vi "Blue Event Log Viewer Main.vi"() -> ()   [LabVIEW 2020, in "Blue Event Log Viewer.lvlib"]
uses:
  Blue Event Log Viewer.lvlib
  <userlib>/Blue Origin/Blue Event Log OpenSource/SubVIs/runlog logging levels.ctl
  <userlib>/Blue Origin/Blue Event Log OpenSource/SubVIs/runlog init options.ctl
  <userlib>/Blue Origin/Blue Event Log OpenSource/SubVIs/VisibleLogLevels.ctl
  <userlib>/Blue Origin/Blue Event Log OpenSource/Classes/RunLog/BlueEventLog.lvclass/BlueEventLog.ctl
  <userlib>/Blue Origin/Blue Event Log OpenSource/Classes/RunLog/Shutdown.vi
  <userlib>/Blue Origin/Blue Event Log OpenSource/SubVIs/Create WaitForFinish Notifier.vi
  <userlib>/Blue Origin/Blue Event Log OpenSource/SubVIs/WaitOn WaitForFinish Notifier.vi
  <userlib>/Blue Origin/Blue Event Log OpenSource/Classes/RunLog/Read Queue Validity.vi
  <vilib>/Utility/error.llb/Clear Errors.vi
  <userlib>/Blue Origin/Blue Event Log OpenSource/Classes/RunLog/New.vi
  <userlib>/Blue Origin/Blue Event Log OpenSource/Classes/RunLog/Stop Load Stream.vi
  <userlib>/Blue Origin/Blue Event Log OpenSource/Classes/RunLog/Clear.vi
  <vilib>/Utility/libraryn.llb/Check if File or Folder Exists.vi
  <vilib>/Utility/file.llb/Is Path and Not Empty.vi
  <vilib>/Utility/libraryn.llb/Librarian Path Location.vi
  <userlib>/_OpenG.lib/file/file.llb/File Exists__ogtk.vi
  <userlib>/_OpenG.lib/file/file.llb/File Exists - Scalar__ogtk.vi
  <userlib>/Blue Origin/Blue Event Log OpenSource/Classes/RunLog/Load log.vi
  <userlib>/Blue Origin/Blue Event Log OpenSource/Classes/RunLog/BlueEventLog.lvclass
  <userlib>/Blue Origin/Blue Event Log OpenSource/BlueEventLog_OpenSource.lvlib
panel:
  in  "Path":path
  in  "poll?":bool=TRUE caption="Poll?"
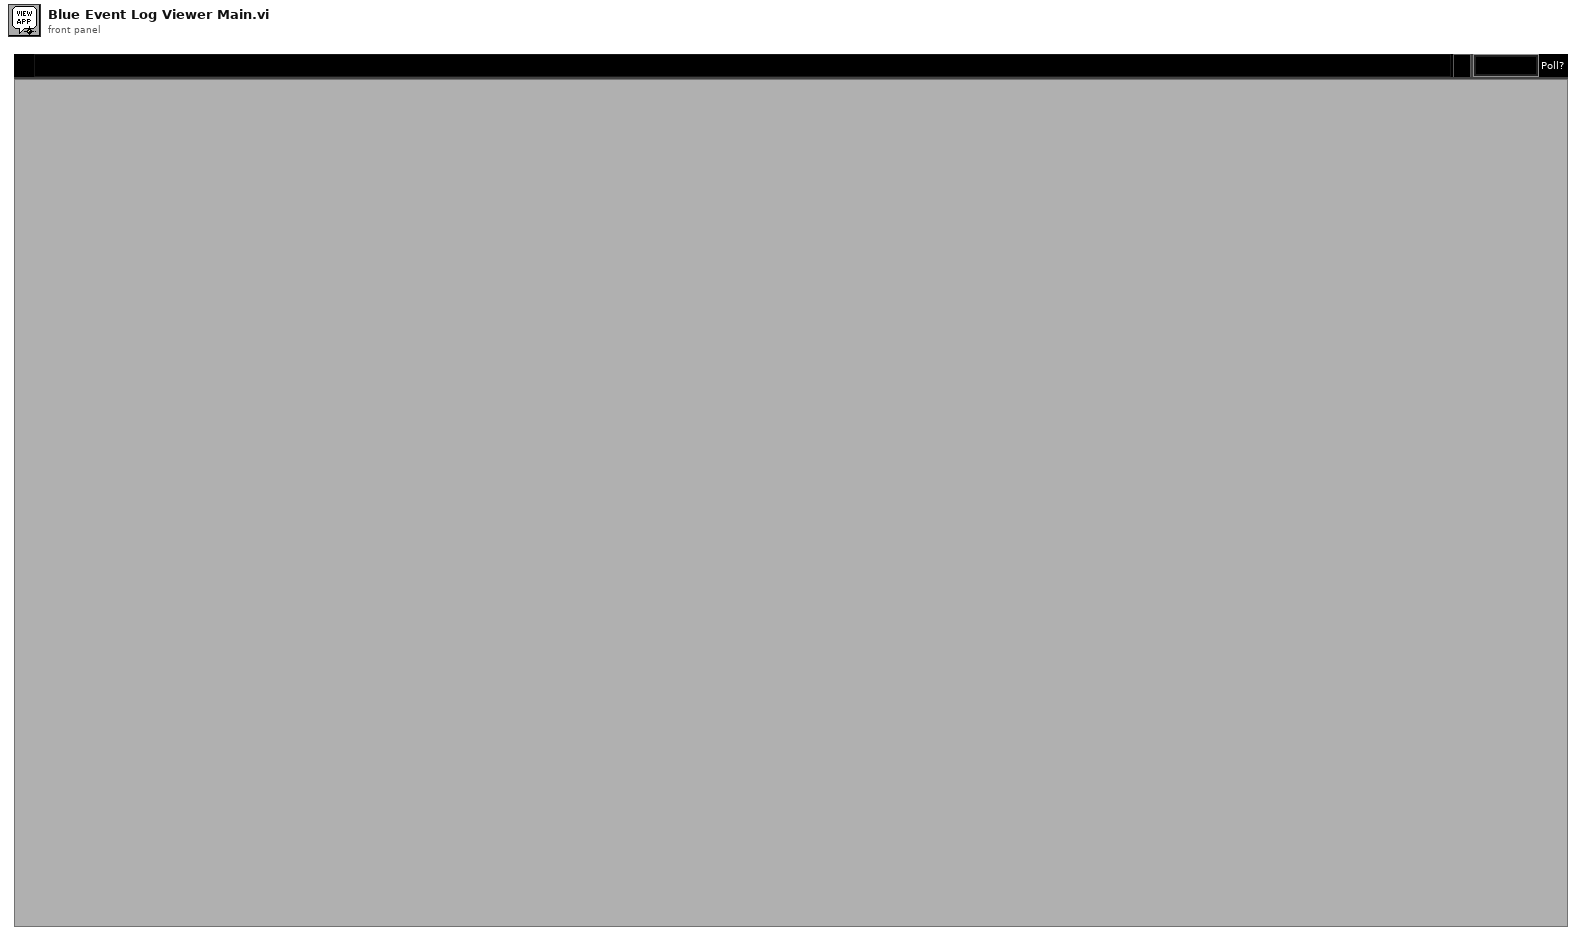
[diagram p1: front panel]
types:
  T1 = typedef "BlueEventLog_OpenSource.lvlib/VisibleLogLevels.ctl" = cluster{"DEBUG":bool, "INFO":bool, "WARNING":bool, "ERROR":bool, "CRITICAL":bool}
  T2 = typedef "BlueEventLog_OpenSource.lvlib/runlog init options.ctl" = cluster{"UI visible? (T)":bool, "Max entry count (10)":i32, "Queue Flush Throttle (100ms)":u32, "Visible Log Levels":T1}
  T3 = typedef "BlueEventLog_OpenSource.lvlib/runlog logging levels.ctl" = enum16{"DEBUG", "INFO", "WARNING", "ERROR", "CRITICAL"}
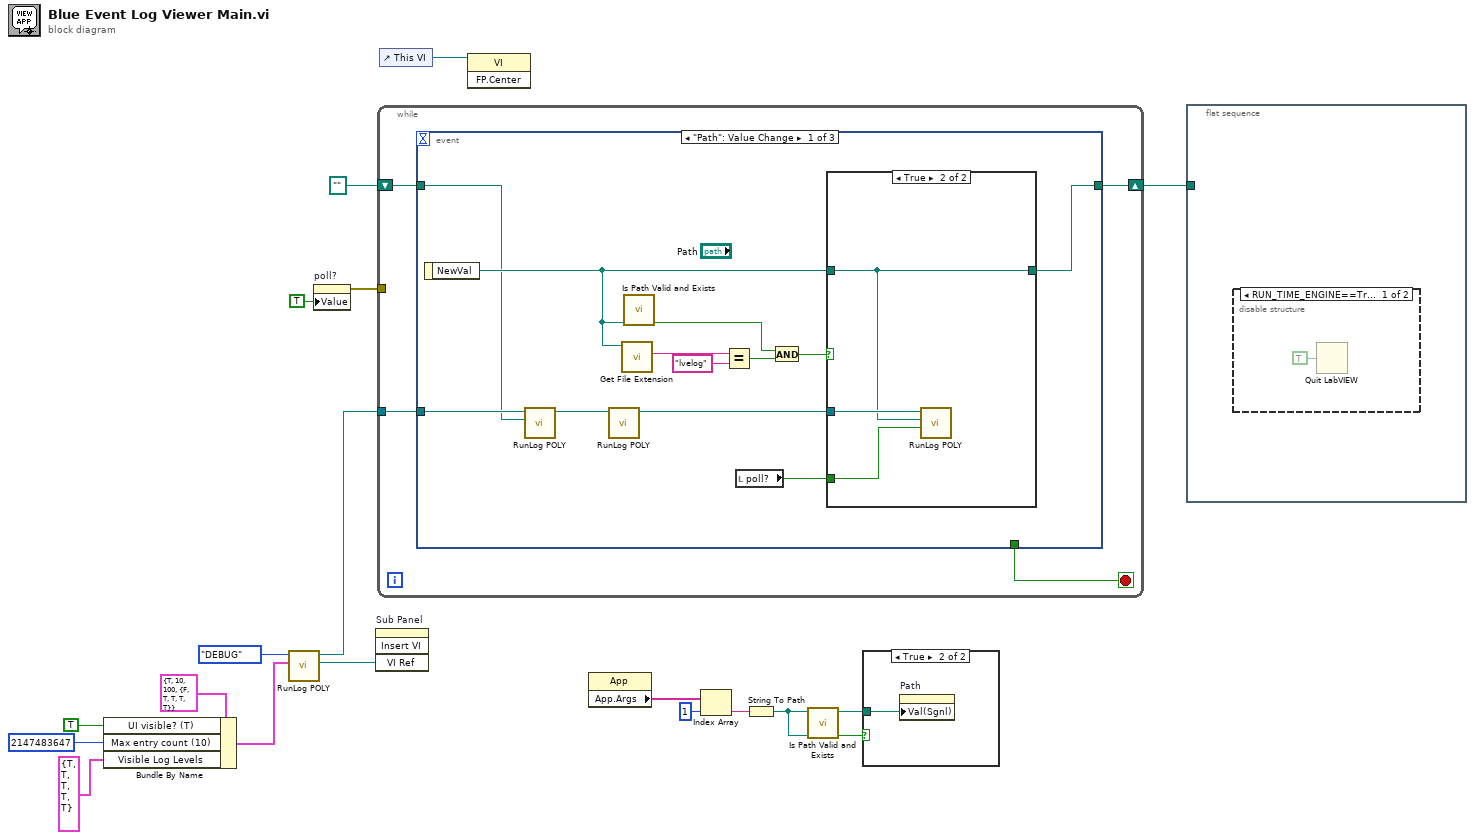
[diagram p0: block diagram]
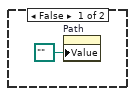
[diagram p3: hidden frame]
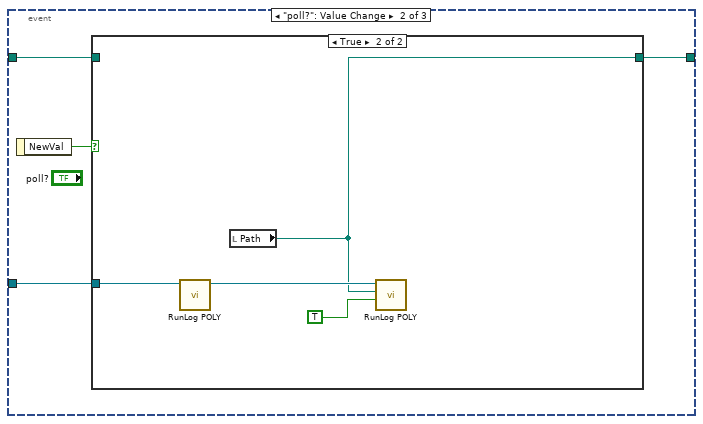
[diagram p5: hidden frame]
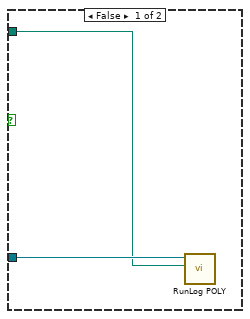
[diagram p6: hidden frame]
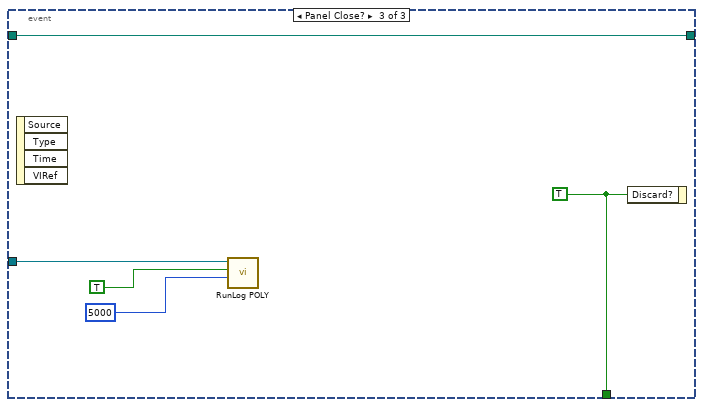
[diagram p7: hidden frame]
diagram:
  n1 = Bundle By Name(cluster=T2 {"UI visible? (T)"=TRUE, "Max entry count (10)"=10, "Queue Flush Throttle (100ms)"=100, "Visible Log Levels"={"DEBUG"=FALSE, "INFO"=TRUE, "WARNING"=TRUE, "ERROR"=TRUE, "CRITICAL"=TRUE}} ("Init options"), "UI visible? (T)"=TRUE, "Max entry count (10)"=2147483647, "Visible Log Levels"=T1 {"DEBUG"=TRUE, "INFO"=TRUE, "WARNING"=TRUE, "ERROR"=TRUE, "CRITICAL"=TRUE}) -> (w3:T2)
  n2 = call-poly <userlib>:"RunLog POLY.vi"("Init options"=w3, "Logging level"=runlog_logging_levels."DEBUG") -> ("VI ref"=w17:refnum<vi>, "Elog out"=w11:refnum<class "BlueEventLog.lvclass">)  [unwired: 7 in, 1 out]
  n3 = property on="poll?" class="Bool (strict)"("Value"=TRUE ("poll?")) -> (error out=w8:errorcluster)  [unwired: 2 in, 1 out]
  n4 = invoke on="Sub Panel" class="SubPnl" method="Insert VI"("VI Ref"=w17) -> ()  [unwired: 3 in, 4 out]
  n5 = while {
    tunnel: w11 -> [w22]
    shift-right: [w20] -> w2
    shift-left: path "" ("NewVal") -> [w21]
    tunnel: w8 -> [_]
    stop <- w19 stop-if-true
    n6 = event shown="[0] \"Path\": Value Change" {
      selector: _ -> [_ _ _]
      dyn-events: _ -> [_ _ _]
      timeout: _ -> [_ _ _]
      tunnel: w22 -> [w27 w41 w50]
      tunnel: w21 -> [w26 w39 w52]
      tunnel: [w23 w38 w52] -> w20
      tunnel: [_ _ w51] -> w19
      event "Path": Value Change {
        n7 = event-data() -> ("NewVal"=w29:path)  [unwired: 1 in]
        n8 = call-poly <userlib>:"RunLog POLY.vi"("log path (*.lvelog)"=w26, "Elog in"=w27) -> ("Elog out"=w25:refnum<class "BlueEventLog.lvclass">)  [unwired: 8 in, 1 out]
        n9 = call-poly <userlib>:"RunLog POLY.vi"("Elog in"=w25) -> ("Elog out"=w24:refnum<class "BlueEventLog.lvclass">)  [unwired: 9 in, 1 out]
        n10 = call <vilib>:"Get File Extension.vi"("file"=w29) -> ("lowercase file extension"=w34:string)  [unwired: 6 in, 4 out]
        n11 = call <userlib>:"Is Path Valid and Exists.vi"("File/Folder Path"=w29) -> ("Valid and Exists?"=w31:bool)  [unwired: 9 in, 1 out]
        n12 = Equal?(x=w34, y="lvelog") -> (x = y?=w32:bool)
        n13 = local read "poll?"() -> (w28:bool)
        n14 = And(x=w31, y=w32) -> (x .and. y?=w30:bool)
        n15 = case shown="True" w30 {
          tunnel: w24 -> [_ w37]
          tunnel: w29 -> [_ w35]
          tunnel: w28 -> [_ w36]
          tunnel: [_ w35] -> w23
          frame False {
          }
          frame True {
            n16 = call-poly <userlib>:"RunLog POLY.vi"("Stream loading? (F)"=w36, "log path (*.lvelog)"=w35, "Elog in"=w37) -> ()  [unwired: 7 in, 2 out]
          }
        }
      }
      event "poll?": Value Change {
        n17 = event-data() -> ("NewVal"=w40:bool)  [unwired: 1 in]
        n18 = case shown="True" w40 {
          tunnel: w41 -> [w43 w47]
          tunnel: w39 -> [w42 _]
          tunnel: [_ w44] -> w38
          frame False {
            n19 = call-poly <userlib>:"RunLog POLY.vi"("log path (*.lvelog)"=w42, "Elog in"=w43) -> ()  [unwired: 8 in, 2 out]
          }
          frame True {
            n20 = call-poly <userlib>:"RunLog POLY.vi"("Elog in"=w47) -> ("Elog out"=w46:refnum<class "BlueEventLog.lvclass">)  [unwired: 9 in, 1 out]
            n21 = local read "Path"() -> (w44:path)
            n22 = call-poly <userlib>:"RunLog POLY.vi"("Stream loading? (F)"=TRUE, "log path (*.lvelog)"=w44, "Elog in"=w46) -> ()  [unwired: 7 in, 2 out]
          }
        }
      }
      event Panel Close? {
        w51 = TRUE ("Discard?")
        n23 = event-data() -> ()  [unwired: 1 in, 4 out]
        n24 = call-poly <userlib>:"RunLog POLY.vi"("wait timeout in ms (-1)"=5000, "Wait until shutdown? (F)"=TRUE, "Elog in"=w50) -> ()  [unwired: 6 in, 3 out]
        n25 = event-data("Discard?"=w51) -> ()  [unwired: 1 in, 1 out]
      }
    }
  }
  n26 = control-ref of="This VI"() -> (w1:refnum<vi>)
  n27 = invoke class="VI" method="FP.Center"(reference=w1) -> ()  [unwired: 2 in, 3 out]
  n28 = property class="App"() -> ("App.Args"=w15:string[])  [unwired: 2 in, 2 out]
  n29 = Index Array(array=w15, index=1) -> (element=w14:string)
  n30 = String To Path(string=w14) -> (path=w12:path)
  n31 = call <userlib>:"Is Path Valid and Exists.vi"("File/Folder Path"=w12) -> ("Valid and Exists?"=w13:bool)  [unwired: 9 in, 1 out]
  n32 = case shown="True" w13 {
    tunnel: w12 -> [_ w54]
    frame False {
      n33 = property on="Path" class="Path"("Value"=path "" ("Path")) -> ()  [unwired: 2 in, 2 out]
    }
    frame True {
      n34 = property on="Path" class="Path"("Val(Sgnl)"=w54) -> ()  [unwired: 2 in, 2 out]
    }
  }
  n35 = flat-sequence {
    tunnel: w2 -> [_]
    frame #0 {
      n36 = disable-structure shown="RUN_TIME_ENGINE==True, Default" {
        frame condition #0 {
          n37 = Quit LabVIEW(quit? (T)=TRUE) -> ()
        }
        frame condition #1 (active) {
        }
      }
    }
  }
